vi "Func_ChangeDataType.vi"(8 "error in (no error)":errorcluster, 9 "Control Path":path, 10 "data type name":string, 11 "template":path=path "C:/Users/dsmith.AMER/Dropbox/CVT Testing/FGV/Template_AllocateMemory.vi") -> (0 "error out":errorcluster, 3 "Final Path":path)   [LabVIEW 2010, in "TemplateGenerator.lvlib"]
uses:
  TemplateGenerator.lvlib
  Current Value Table.lvlib
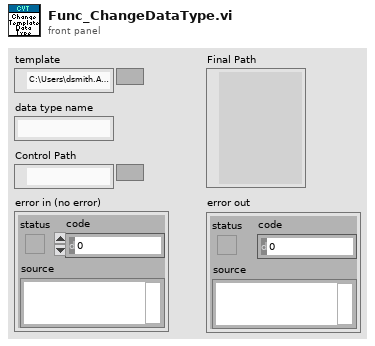
[diagram p1: front panel]
types:
  T1 = enum32{"Invalid", "Standard", "Closed", "Hidden", "Minimized", "Maximized"}
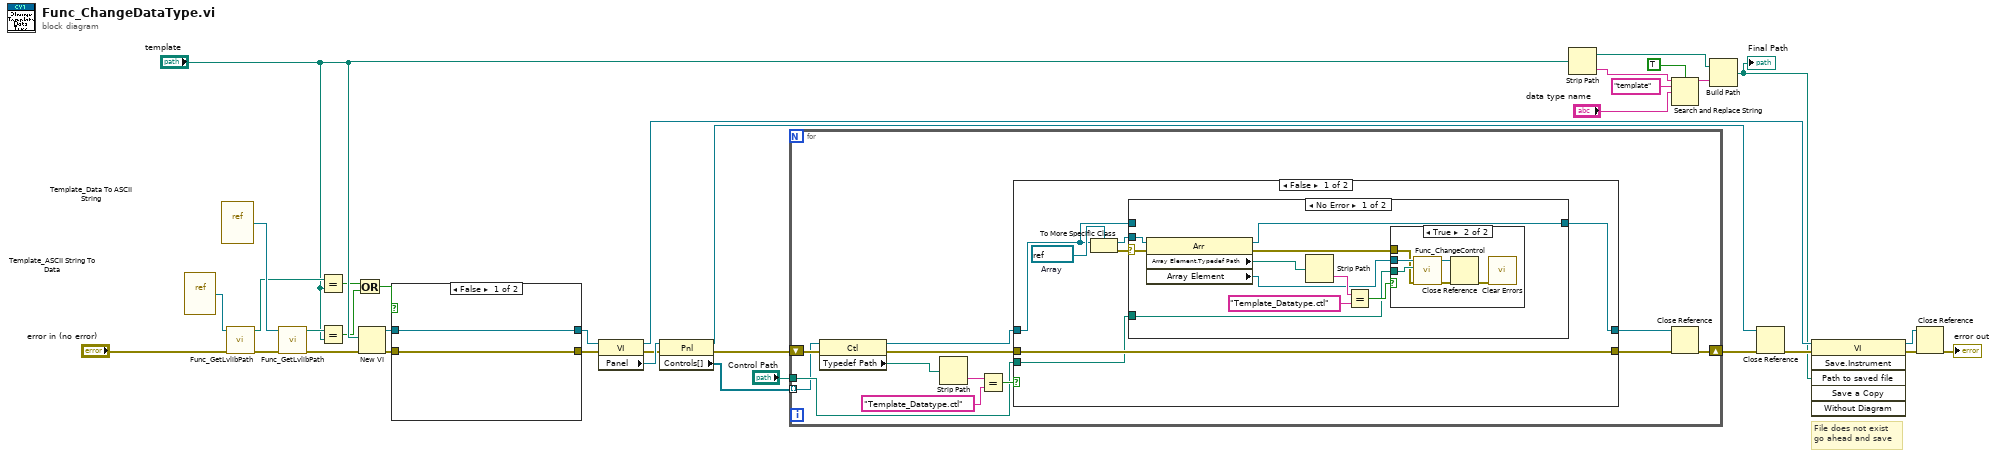
[diagram p0: block diagram]
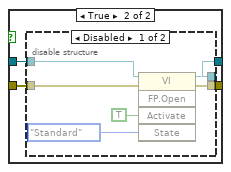
[diagram p2: hidden frame]
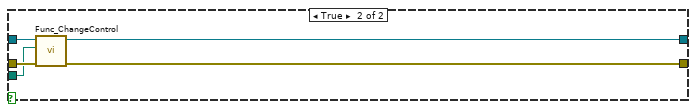
[diagram p6: hidden frame]
diagram:
  # "File does not exist\ngo ahead and save"
  n1 = vi-ref "Template_ASCII String To Data.vi"() -> (w14:refnum<vi>)
  n2 = vi-ref "Template_Data To ASCII String.vi"() -> (w15:refnum<vi>)
  n3 = call "Func_GetLvlibPath.vi"("error in (no error)"="error in (no error)", "VI in"=w14) -> ("error out"=w13:errorcluster, "VI Path"=w12:path)  [unwired: 8 in]
  n4 = call "Func_GetLvlibPath.vi"("error in (no error)"=w13, "VI in"=w15) -> ("error out"=w7:errorcluster, "VI Path"=w11:path)  [unwired: 8 in]
  n5 = Equal?(x=w12, y="template") -> (x = y?=w9:bool)
  n6 = Equal?(x=w11, y="template") -> (x = y?=w8:bool)
  n7 = Or(x=w9, y=w8) -> (x .or. y?=w1:bool)
  n8 = New VI(8:w7, 10:"template") -> (0:w4:errorcluster, 3:w5:refnum<vi>)  [unwired: 5 in]
  n9 = case shown="False" w1 {
    tunnel: w5 -> [w36 w40]
    tunnel: w4 -> [w35 w39]
    tunnel: [w36 w38] -> w3
    tunnel: [w35 w37] -> w2
    frame False {
    }
    frame True {
      n10 = disable-structure shown="Disabled" {
        disable-tunnel: w40 -> [w46 w48]
        disable-tunnel: w39 -> [w45 w47]
        disable-tunnel: [w44 w48] -> w38
        disable-tunnel: [w43 w47] -> w37
        frame Disabled {
          n11 = invoke class="VI" method="FP.Open"(reference=w46, error in=w45, "Activate"=TRUE ("Activate?"), "State"=T1."Standard") -> (reference out=w44:refnum<vi>, error out=w43:errorcluster)  [unwired: 1 in, 3 out]
        }
        frame Enabled {
        }
      }
    }
  }
  n12 = property class="VI"(reference=w3, error in=w2) -> (reference out=w27:refnum<vi>, error out=w32:errorcluster, "Panel"=w34:refnum<vi>)
  n13 = property class="Pnl"(reference=w34, error in=w32) -> (reference out=w28:refnum<vi>, error out=w31:errorcluster, "Controls[]"=w33:refnum<vi>[])
  n14 = for {
    tunnel: w33 -> [w50] mode=indexing
    shift-right: [w55] -> w30
    shift-left: w31 -> [w59]
    tunnel: "Control Path" -> [w51]
    n15 = property class="Ctl"(reference=w50, error in=w59) -> (reference out=w49:refnum<vi>, error out=w58:errorcluster, "Typedef Path"=w54:path)
    n16 = Strip Path(path=w54) -> (name=w53:string)  [unwired: 1 out]
    n17 = Equal?(x=w53, y="Template_Datatype.ctl") -> (x = y?=w60:bool)
    n18 = case shown="False" w60 {
      tunnel: w49 -> [w62 w89]
      tunnel: w58 -> [w64 w88]
      tunnel: [w63 w85] -> w57
      tunnel: [w64 w86] -> w56
      tunnel: w51 -> [w61 w87]
      frame False {
        w67 = refnum<vi> refnum  # Array
        n19 = To More Specific Class(target class=w67, reference=w62) -> (specific class reference=w65:refnum<vi>, error out=w66:errorcluster)  [unwired: 1 in]
        n20 = case shown="No Error" w66 {
          selector: w66 -> [w69 _]
          tunnel: w65 -> [w77 _]
          tunnel: [w71 w84] -> w63
          tunnel: w62 -> [_ w84]
          tunnel: w61 -> [w68 _]
          frame No Error {
            n21 = property class="Arr"(reference=w77, error in=w69) -> (reference out=w71:refnum<vi>, error out=w70:errorcluster, "Array Element.Typedef Path"=w76:path, "Array Element"=w72:refnum<vi>)
            n22 = Strip Path(path=w76) -> (name=w74:string)  [unwired: 1 out]
            n23 = Equal?(x=w74, y="Template_Datatype.ctl") -> (x = y?=w73:bool)
            n24 = case shown="True" w73 {
              tunnel: w72 -> [_ w81]
              tunnel: w70 -> [_ w78]
              tunnel: w68 -> [_ w82]
              frame False {
              }
              frame True {
                n25 = call "Func_ChangeControl.vi"("error in (no error)"=w78, "Control Path"=w82, "Control in"=w81) -> ("error out"=w79:errorcluster, "GObject out"=w80:refnum<vi>)  [unwired: 7 in]
                n26 = Close Reference(reference=w80, error in (no error)=w79) -> (error out=w83:errorcluster)
                n27 = call <vilib>:"Clear Errors.vi"("error in (no error)"=w83) -> ()  [unwired: 6 in, 1 out]
              }
            }
          }
          frame Error {
          }
        }
      }
      frame True {
        n28 = call "Func_ChangeControl.vi"("error in (no error)"=w88, "Control Path"=w87, "Control in"=w89) -> ("error out"=w86:errorcluster, "GObject out"=w85:refnum<vi>)  [unwired: 7 in]
      }
    }
    n29 = Close Reference(reference=w57, error in (no error)=w56) -> (error out=w55:errorcluster)
  }
  n30 = Strip Path(path="template") -> (stripped path=w16:path, name=w24:string)
  n31 = Search and Replace String(case sensitive?=TRUE ("ignore case? (F)"), input string=w24, search string="template", replace string="data type name") -> (result string=w20:string)  [unwired: 4 in, 3 out]
  n32 = Build Path(base path=w16, name or relative path=w20) -> (appended path=w19:path)
  "Final Path" <- w19
  n33 = Close Reference(reference=w28, error in (no error)=w30) -> (error out=w29:errorcluster)
  n34 = invoke class="VI" method="Save.Instrument"(reference=w27, error in=w29, "Path to saved file"=w19) -> (reference out=w25:refnum<vi>, error out=w26:errorcluster)  [unwired: 3 in, 4 out]
  n35 = Close Reference(reference=w25, error in (no error)=w26) -> (error out=→"error out":errorcluster)
